vi "Get Digital Project Directory.vi"(11 "error in (no error)":errorcluster) -> (4 "Digital Project Directory":path, 15 "error out":errorcluster)   [LabVIEW 2018, in "MIPI RFFE API.lvlib"]
uses:
  MIPI RFFE API.lvlib
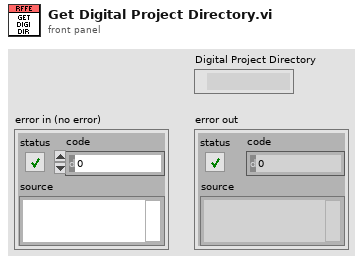
[diagram p1: front panel]
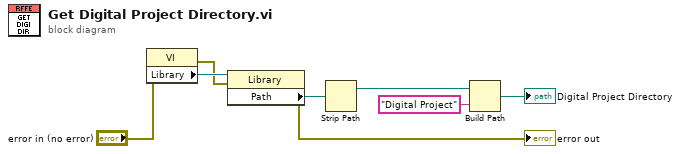
[diagram p0: block diagram]
diagram:
  n1 = property on="Property Node" class="VI"(error in="error in (no error)") -> (error out=w2:errorcluster, "Library"=w6:refnum<vi>)  [unwired: 1 in, 1 out]
  n2 = property on="Property Node" class="Library"(reference=w6, error in=w2) -> (error out=→"error out":errorcluster, "Path"=w7:path)  [unwired: 1 out]
  n3 = Strip Path(path=w7) -> (stripped path=w5:path)  [unwired: 1 out]
  n4 = Build Path(base path=w5, name or relative path="Digital Project") -> (appended path=→"Digital Project Directory":path)
